vi "Generate Image.vi"(11 "Grid.lvclass":refnum<class "Grid.lvclass">) -> (3 "new picture":picture)   [LabVIEW 2016, in "Grid.lvclass"]
uses:
  Grid.lvclass
  <vilib>/picture/picture.llb/Draw True-Color Pixmap.vi
  Pixel/Pixel.lvclass
panel:
  in  "Color Array":u32[](array[colorbox])=[16711680, 16448250, 16860]
  out "Numeric 2":i32
  out "Color Box":u32(colorbox)
  out "Numeric":i32
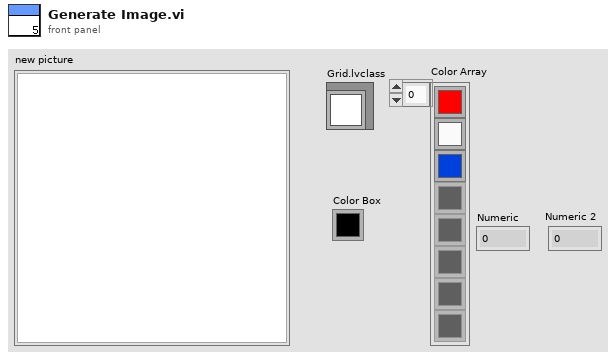
[diagram p1: front panel]
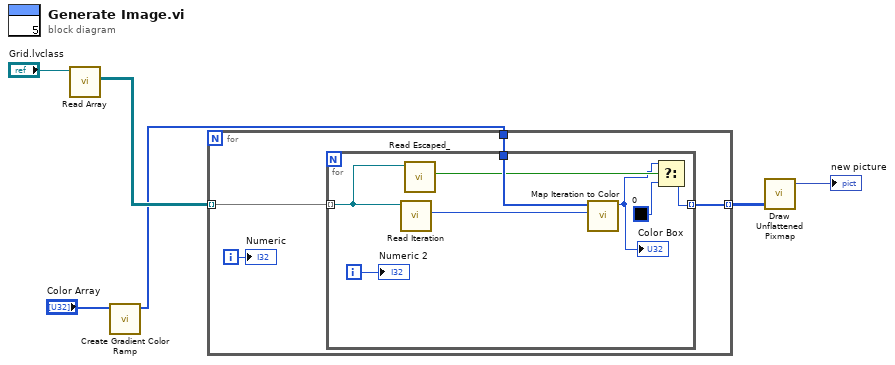
[diagram p0: block diagram]
diagram:
  n1 = call-dynamic "Read Array.vi"("Grid in"="Grid.lvclass") -> ("Grid"=w5:refnum<class "Pixel.lvclass">[][])  [unwired: 8 in, 2 out]
  n2 = call "Create Gradient Color Ramp.vi"("Color Array"="Color Array") -> ("Color Table"=w1:u32[])  [unwired: 8 in, 2 out]
  n3 = for {
    tunnel: w5 -> [w10] mode=indexing
    tunnel: w1 -> [w9]
    tunnel: [w8] -> w3 mode=indexing
    i -> [w7]
    n4 = for {
      tunnel: w10 -> [w16] mode=indexing
      tunnel: w9 -> [w18]
      tunnel: [w14] -> w8 mode=indexing
      i -> [w17]
      n5 = call-dynamic "Read Iteration.vi"("Pixel in"=w16) -> ("Iteration"=w13:u16)  [unwired: 8 in, 2 out]
      n6 = call-dynamic "Read Escaped_ .vi"("Pixel in"=w16) -> ("Escaped?"=w15:bool)  [unwired: 8 in, 2 out]
      n7 = call "Map Iteration to Color.vi"("Iteration"=w13, "Color Table"=w18) -> ("element"=w11:u32)  [unwired: 9 in]
      "Color Box" <- w11
      n8 = Select(t=w11, s=w15, f=u32 0 ("Color Box 2")) -> (s? t:f=w14:u32)
      "Numeric 2" <- w17
    }
    "Numeric" <- w7
  }
  n9 = call-poly <vilib>:"Draw Unflattened Pixmap.vi"("data (RGB format)"=w3) -> ("new picture"=→"new picture":picture)  [unwired: 8 in]
